vi "Verify Type.vi"(8 "error in (no error)":errorcluster, 11 "CIF_CIPC_Fifo_U8 in":refnum<class "CIF_CIPC_Fifo_DAQ.lvclass">) -> (0 "error out":errorcluster, 3 "CIF_CIPC_Fifo_U8 out":refnum<class "CIF_CIPC_Fifo_DAQ.lvclass">)   [LabVIEW 2021, in "CIF_CIPC_Fifo_DAQ.lvclass"]
uses:
  CIF_CIPC_Fifo_DAQ.lvclass
  D:/dev/Packages/CIF_Channels_Core/src/CIPC_Channels/CIF_CIPC_Chan/CIF_CIPC_Chn.lvclass
  D:/dev/Packages/CIF_Channels_Core/src/CIFChannels/CIFChannels.lvclass
  CIF_CIPC_Chan/CIF_CIPC_Chn.lvclass/CIF_CIPC_Chn.ctl
  CIFChannels/CIFChannels.lvclass/CIFChannels.ctl
  CIF_CIPC_Chan/Typedef/CIPC Channel Error.ctl
  <vilib>/CIF Foundation/CIF CIPC/SubVIs/Check Error.vi
  <vilib>/CIF Foundation/CIF CIPC/SubVIs/Get dll Path.vi
  <vilib>/CIF Foundation/CIF Utilities/Errors/Append Error Location.vi
  <vilib>/Utility/error.llb/Trim Whitespace.vi
  <vilib>/Utility/error.llb/Error Cluster From Error Code.vi
  CIF_CIPC_Chan/CIF_CIPC_Chn.lvclass
  CIFChannels/CIFChannels.lvclass
  <vilib>/CIF Foundation/CIF CIPC/CIF_NI_CIPC.lvlib
  <vilib>/CIF Foundation/CIF Utilities/DataTypes/DataTypes_CIF_U.lvlib
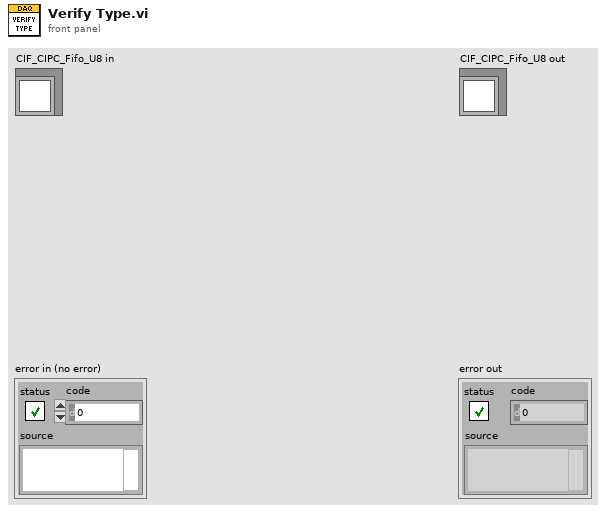
[diagram p1: front panel]
types:
  T1 = typedef "CIF_CIPC_Chn.lvclass/CIPC Channel Error.ctl" = enum16{"Type Mismatch"}
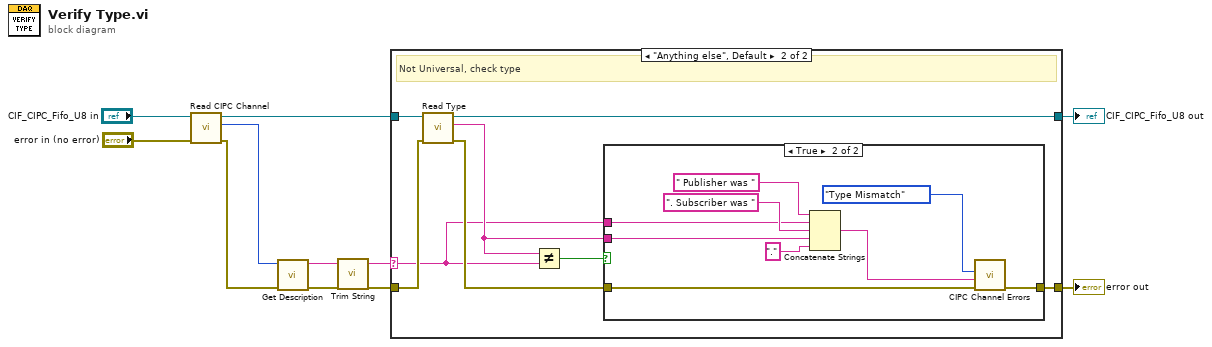
[diagram p0: block diagram]
diagram:
  n1 = call "Read CIPC Channel.vi"("error in (no error)"="error in (no error)", "CIFTag in"="CIF_CIPC_Fifo_U8 in") -> ("error out"=w6:errorcluster, "CIPC Channel"=w8:u64, "CIFTag out"=w9:refnum<class "CIF_CIPC_Fifo_DAQ.lvclass">)  [unwired: 7 in]
  n2 = call <vilib>:"Get Description.vi"("error in (no error)"=w6, "CIPC Reference"=w8) -> ("error out"=w5:errorcluster, "Description"=w2:string)  [unwired: 8 in]
  n3 = call <vilib>:"Trim String.vi"("String in"=w2) -> ("Trimmed String"=w1:string)  [unwired: 4 in]
  n4 = case shown="\"Anything else\", Default" w1 {
    selector: w1 -> [_ w13]
    tunnel: w9 -> [w12 w20]
    tunnel: w5 -> [w11 w19]
    tunnel: [w11 w17] -> w4
    tunnel: [w12 w16] -> w3
    frame "CIF_CIPC_Universal" {
      # "Universal skips this check"
    }
    frame "Anything else", Default {
      # "Not Universal, check type"
      n5 = call "Read Type.vi"("error in (no error)"=w19, "CIFChannels in"=w20) -> ("error out"=w18:errorcluster, "Type"=w14:string, "CIFChannels out"=w16:refnum<class "CIF_CIPC_Fifo_DAQ.lvclass">)  [unwired: 7 in]
      n6 = Not Equal?(x=w14, y=w13) -> (x != y?=w15:bool)
      n7 = case shown="True" w15 {
        tunnel: w18 -> [w21 w29]
        tunnel: [w21 w28] -> w17
        tunnel: w13 -> [_ w22]
        tunnel: w14 -> [_ w25]
        frame False {
        }
        frame True {
          n8 = Concatenate Strings(" Publisher was ", w22, ". Subscriber was ", w25, ".") -> (w23:string)
          n9 = call "CIPC Channel Errors.vi"("error in (no error)"=w29, "String to Append"=w23, "Error"=CIPC_Channel_Error."Type Mismatch") -> ("error out"=w28:errorcluster)  [unwired: 8 in]
        }
      }
    }
  }
  "error out" <- w4
  "CIF_CIPC_Fifo_U8 out" <- w3
